vi "IPS magnet power supply - send GPIB cmd.vi"(8 "error in (no error)":errorcluster, 10 "Cmd string":string="setfield 0.12345") -> (0 "error out":errorcluster={"status"=FALSE, "code"=1073676293, "source"="VISA Read in IPS magnet power supply - send GPIB cmd.vi"}, 2 "Response":string="J\r")   [LabVIEW 2019]
doc: "Nicolas Weiss - EPFL - IPHYS 2019\n----\nThis VI sends the GPIB commands to the device (without performing syntax and in-range argument check).\nThus, the commands *must* first be checked by the \"Check and send command to corresponding device.vi\""
uses:
  _Global variables 1.vi
panel:
  out "Arguments":string[](array[string])=["0.12345"]
  # "IPSheater on\nFieldRate 0.05\nFieldSetpoint 0.05\nGetFieldSetpoint\nToFieldSetpoint\nGetField\nHoldField\nToZeroField\nIPSstatus"
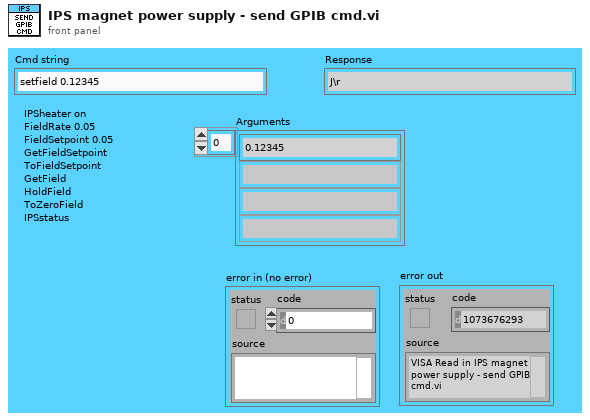
[diagram p1: front panel]
types:
  T1 = cluster{"[0]":i32, "[1]":i32, "[2]":i32, "[3]":i32, "[4]":i32, "[5]":i32, "[6]":i32, "[7]":i32, "[8]":i32}
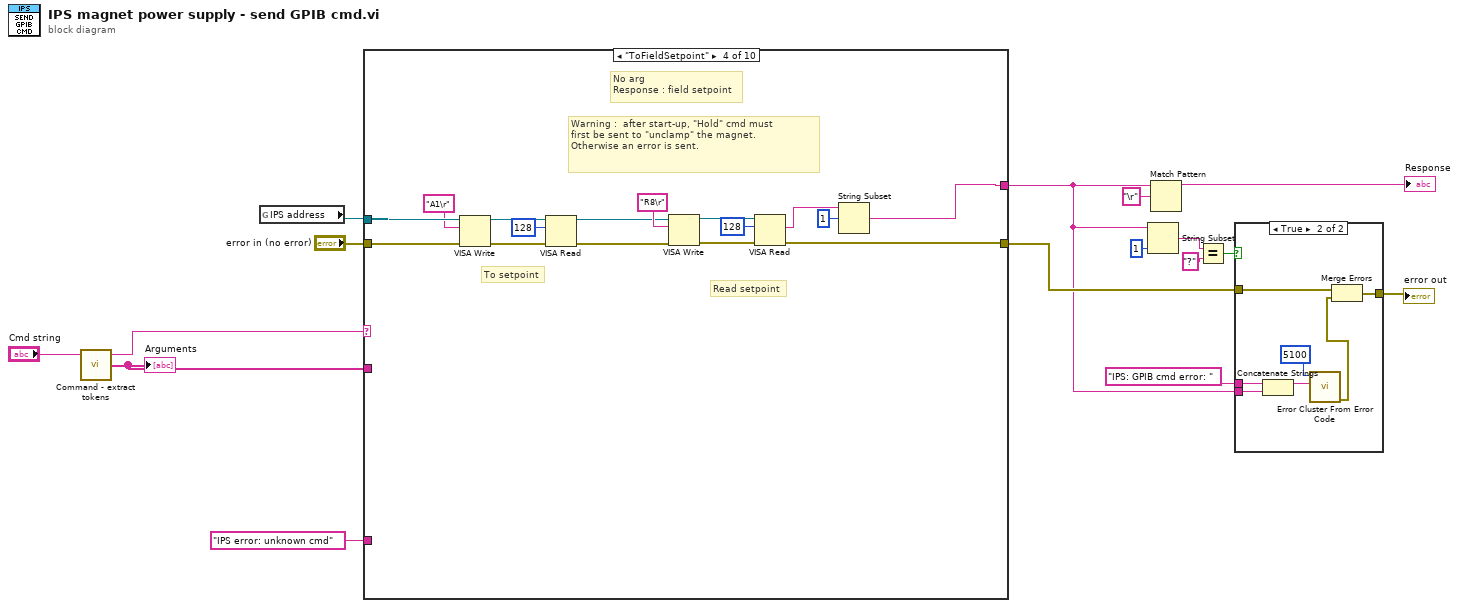
[diagram p0: block diagram]
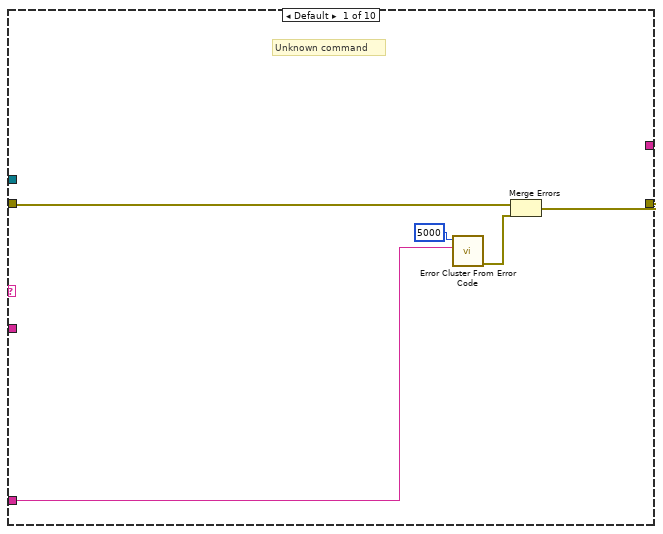
[diagram p3: hidden frame]
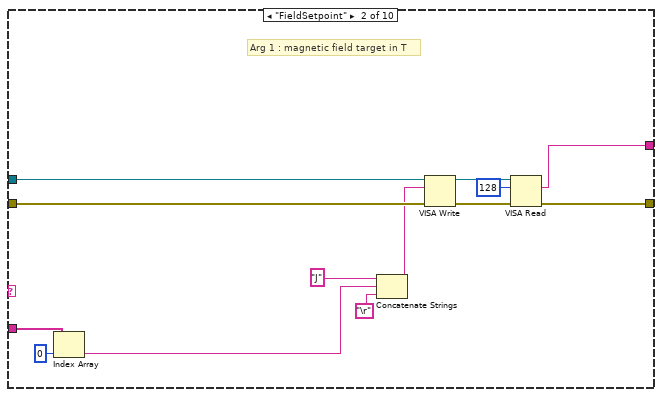
[diagram p4: hidden frame]
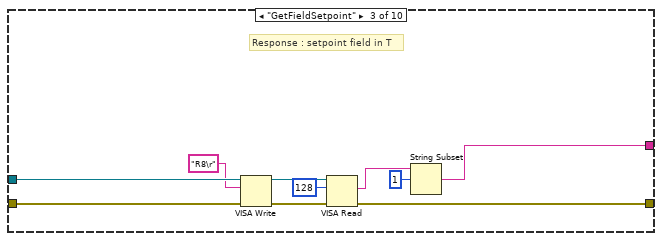
[diagram p5: hidden frame]
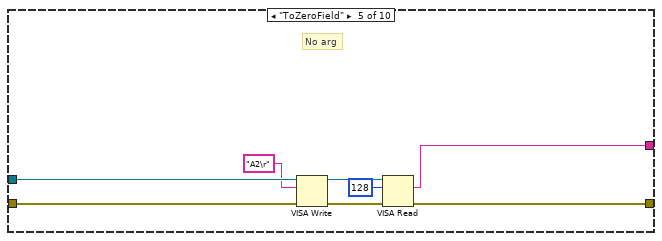
[diagram p6: hidden frame]
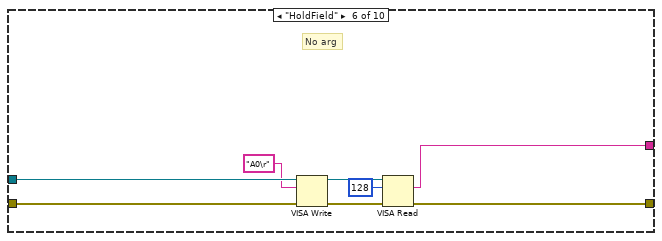
[diagram p7: hidden frame]
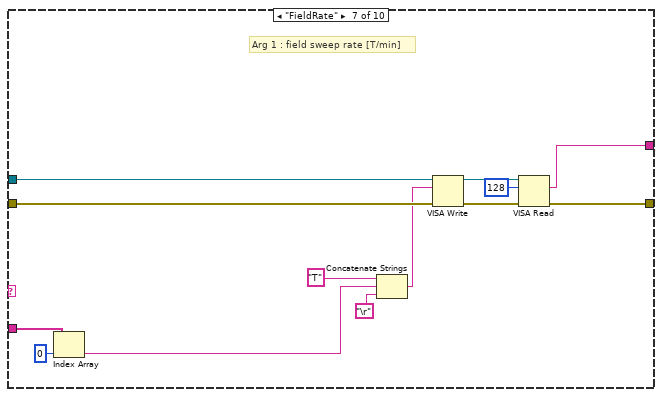
[diagram p8: hidden frame]
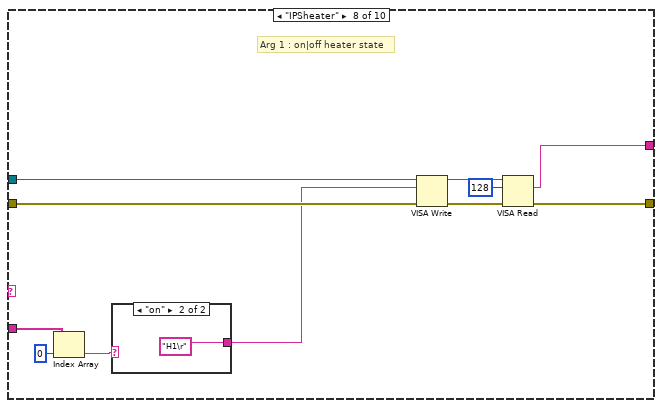
[diagram p9: hidden frame]
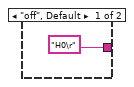
[diagram p10: hidden frame]
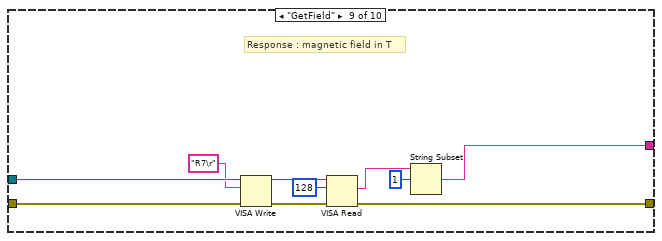
[diagram p11: hidden frame]
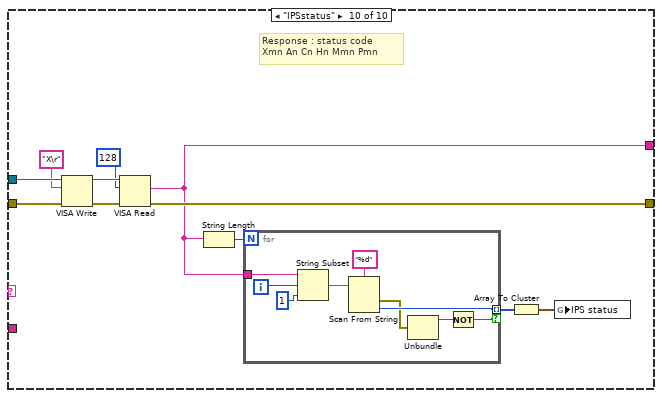
[diagram p12: hidden frame]
diagram:
  n1 = call "Command - extract tokens.vi"("Cmd string"="Cmd string") -> ("Arguments"=w13:string[], "Command"=w11:string)  [unwired: 2 in, 1 out]
  "Arguments" <- w13
  n2 = global read "_Global variables 1.vi" "IPS address"() -> (w15:refnum<visa-resource-name>)
  n3 = case shown="\"ToFieldSetpoint\"" w11 {
    tunnel: w13 -> [_ w33 _ _ _ _ w88 w99 _ _]
    tunnel: w15 -> [_ w31 w43 w59 w67 w75 w86 w97 w111 w122]
    tunnel: "error in (no error)" -> [w18 w32 w44 w60 w68 w76 w87 w98 w112 w123]
    tunnel: [w19 w22 w39 w46 w62 w70 w77 w92 w107 w118] -> w4
    tunnel: "IPS error: unknown cmd" ("format string") -> [w17 _ _ _ _ _ _ _ _ _]
    tunnel: [_ w25 w35 w45 w65 w73 w80 w95 w103 w113] -> w1
    frame Default {
      # "Unknown command"
      n4 = call <vilib>:"Error Cluster From Error Code.vi"("error message (\"\")"=w17, "error code (0)"=5000) -> ("error out"=w21:errorcluster)  [unwired: 7 in]
      n5 = Merge Errors(w18, w21) -> (w19:errorcluster)
    }
    frame "FieldSetpoint" {
      # "Arg 1 : magnetic field target in T"
      n6 = Index Array(array=w33, index=0) -> (element=w29:string)
      n7 = Concatenate Strings("J" ("format string"), w29, "\r") -> (w28:string)
      n8 = VISA Write(VISA resource name=w31, write buffer=w28, error in (no error)=w32) -> (VISA resource name out=w26:refnum<visa-resource-name>, error out=w23:errorcluster)  [unwired: 1 out]
      n9 = VISA Read(VISA resource name=w26, byte count=u32 128, error in (no error)=w23) -> (read buffer=w25:string, error out=w22:errorcluster)  [unwired: 2 out]
    }
    frame "GetFieldSetpoint" {
      # "Response : setpoint field in T"
      n10 = VISA Write(VISA resource name=w43, write buffer="R8\r" ("format string"), error in (no error)=w44) -> (VISA resource name out=w42:refnum<visa-resource-name>, error out=w40:errorcluster)  [unwired: 1 out]
      n11 = VISA Read(VISA resource name=w42, byte count=u32 128, error in (no error)=w40) -> (read buffer=w37:string, error out=w39:errorcluster)  [unwired: 2 out]
      n12 = String Subset(string=w37, offset (0)=1) -> (substring=w35:string)  [unwired: 1 in]
    }
    frame "ToFieldSetpoint" {
      # "Read setpoint"
      # "To setpoint"
      # "Warning :  after start-up, \"Hold\" cmd must\nfirst be sent to \"unclamp\" the magnet.\nOtherwise an error is sent."
      # "No arg\nResponse : field setpoint"
      n13 = VISA Write(VISA resource name=w59, write buffer="A1\r" ("format string"), error in (no error)=w60) -> (VISA resource name out=w58:refnum<visa-resource-name>, error out=w56:errorcluster)  [unwired: 1 out]
      n14 = VISA Read(VISA resource name=w58, byte count=u32 128, error in (no error)=w56) -> (VISA resource name out=w47:refnum<visa-resource-name>, error out=w48:errorcluster)  [unwired: 2 out]
      n15 = VISA Write(VISA resource name=w47, write buffer="R8\r" ("format string"), error in (no error)=w48) -> (VISA resource name out=w54:refnum<visa-resource-name>, error out=w53:errorcluster)  [unwired: 1 out]
      n16 = VISA Read(VISA resource name=w54, byte count=u32 128, error in (no error)=w53) -> (read buffer=w52:string, error out=w46:errorcluster)  [unwired: 2 out]
      n17 = String Subset(string=w52, offset (0)=1) -> (substring=w45:string)  [unwired: 1 in]
    }
    frame "ToZeroField" {
      # "No arg"
      n18 = VISA Write(VISA resource name=w67, write buffer="A2\r" ("format string"), error in (no error)=w68) -> (VISA resource name out=w66:refnum<visa-resource-name>, error out=w63:errorcluster)  [unwired: 1 out]
      n19 = VISA Read(VISA resource name=w66, byte count=u32 128, error in (no error)=w63) -> (read buffer=w65:string, error out=w62:errorcluster)  [unwired: 2 out]
    }
    frame "HoldField" {
      # "No arg"
      n20 = VISA Write(VISA resource name=w75, write buffer="A0\r" ("format string"), error in (no error)=w76) -> (VISA resource name out=w74:refnum<visa-resource-name>, error out=w71:errorcluster)  [unwired: 1 out]
      n21 = VISA Read(VISA resource name=w74, byte count=u32 128, error in (no error)=w71) -> (read buffer=w73:string, error out=w70:errorcluster)  [unwired: 2 out]
    }
    frame "FieldRate" {
      # "Arg 1 : field sweep rate [T/min]"
      n22 = Index Array(array=w88, index=0) -> (element=w84:string)
      n23 = Concatenate Strings("T" ("format string"), w84, "\r") -> (w83:string)
      n24 = VISA Write(VISA resource name=w86, write buffer=w83, error in (no error)=w87) -> (VISA resource name out=w81:refnum<visa-resource-name>, error out=w78:errorcluster)  [unwired: 1 out]
      n25 = VISA Read(VISA resource name=w81, byte count=u32 128, error in (no error)=w78) -> (read buffer=w80:string, error out=w77:errorcluster)  [unwired: 2 out]
    }
    frame "IPSheater" {
      # "Arg 1 : on|off heater state"
      n26 = Index Array(array=w99, index=0) -> (element=w91:string)
      n27 = case shown="\"on\"" w91 {
        tunnel: ["H0\r" ("format string") "H1\r" ("format string")] -> w90
        frame "off", Default {
        }
        frame "on" {
        }
      }
      n28 = VISA Write(VISA resource name=w97, write buffer=w90, error in (no error)=w98) -> (VISA resource name out=w96:refnum<visa-resource-name>, error out=w93:errorcluster)  [unwired: 1 out]
      n29 = VISA Read(VISA resource name=w96, byte count=u32 128, error in (no error)=w93) -> (read buffer=w95:string, error out=w92:errorcluster)  [unwired: 2 out]
    }
    frame "GetField" {
      # "Response : magnetic field in T"
      n30 = VISA Write(VISA resource name=w111, write buffer="R7\r" ("format string"), error in (no error)=w112) -> (VISA resource name out=w110:refnum<visa-resource-name>, error out=w108:errorcluster)  [unwired: 1 out]
      n31 = VISA Read(VISA resource name=w110, byte count=u32 128, error in (no error)=w108) -> (read buffer=w105:string, error out=w107:errorcluster)  [unwired: 2 out]
      n32 = String Subset(string=w105, offset (0)=1) -> (substring=w103:string)  [unwired: 1 in]
    }
    frame "IPSstatus" {
      # "Response : status code\nXmn An Cn Hn Mmn Pmn"
      n33 = VISA Write(VISA resource name=w122, write buffer="X\r" ("format string"), error in (no error)=w123) -> (VISA resource name out=w121:refnum<visa-resource-name>, error out=w119:errorcluster)  [unwired: 1 out]
      n34 = VISA Read(VISA resource name=w121, byte count=u32 128, error in (no error)=w119) -> (read buffer=w113:string, error out=w118:errorcluster)  [unwired: 2 out]
      n35 = String Length(string=w113) -> (length=w116:i32)
      n36 = for {
        N: w116 -> [_]
        tunnel: w113 -> [w132]
        tunnel: [w127] -> w115 mode=indexing if=w124
        i -> [w131]
        n37 = String Subset(string=w132, offset (0)=w131, length (rest)=1 ("length (rest)")) -> (substring=w130:string)
        n38 = Scan From String(format string="%d", input string=w130) -> (error out=w126:errorcluster, output 1=w127:i32)  [unwired: 3 in, 2 out]
        n39 = Unbundle(w126) -> ("status"=w125:bool)  [unwired: 2 out]
        n40 = Not(x=w125) -> (.not. x?=w124:bool)
      }
      n41 = Array To Cluster(array=w115) -> (cluster=w114:T1)
      n42 = global write "_Global variables 1.vi" "IPS status"(w114) -> ()
    }
  }
  n43 = String Subset(string=w1, length (rest)=1 ("length (rest)")) -> (substring=w7:string)  [unwired: 1 in]
  n44 = Match Pattern(string=w1, regular expression="\r") -> (before substring=→"Response":string)  [unwired: 1 in, 3 out]
  n45 = Equal?(x=w7, y="?" ("regular expression")) -> (x = y?=w5:bool)
  n46 = case shown="True" w5 {
    tunnel: w4 -> [w133 w139]
    tunnel: "IPS: GPIB cmd error: " ("format string") -> [_ w136]
    tunnel: [w133 w137] -> w2
    tunnel: w1 -> [_ w134]
    frame False {
    }
    frame True {
      n47 = Concatenate Strings(w136, w134) -> (w135:string)
      n48 = call <vilib>:"Error Cluster From Error Code.vi"("error message (\"\")"=w135, "error code (0)"=5100) -> ("error out"=w138:errorcluster)  [unwired: 7 in]
      n49 = Merge Errors(w139, w138) -> (w137:errorcluster)
    }
  }
  "error out" <- w2
